vi "Library Path.vi"() -> (0 "Library Path":path=path "C:/LQ/bin/LQ.dll")   [LabVIEW 2014, in "LQ Core.lvlib"]
uses:
  LQ Core.lvlib
  <vilib>/Utility/sysdir.llb/System Directory Type.ctl
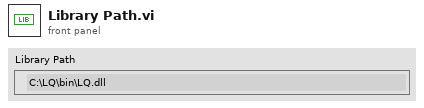
[diagram p1: front panel]
types:
  T1 = typedef "System Directory Type.ctl" = i32
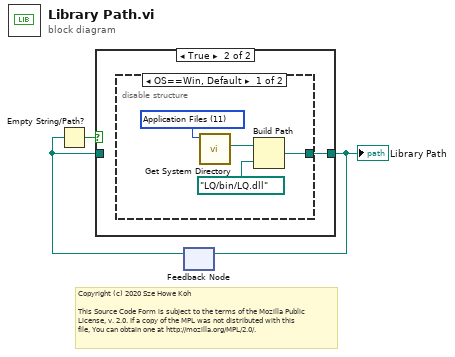
[diagram p0: block diagram]
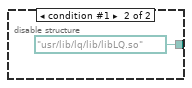
[diagram p3: hidden frame]
diagram:
  # "Copyright (c) 2020 Sze Howe Koh\n\nThis Source Code Form is subject to the terms of the Mozilla Public\nLicense, v. 2.0. If a copy of the MPL was not distributed with this\nfile, You can obtain one at http://mozilla.org/MPL/2.0/."
  n1 = feedback #1() -> (w2:path)  [unwired: 1 in]
  n2 = Empty String/Path?(string/path=w2) -> (empty?=w3:bool)
  n3 = case shown="True" w3 {
    tunnel: [w4 w5] -> w1
    tunnel: w2 -> [w4 _]
    frame False {
    }
    frame True {
      n4 = disable-structure shown="OS==Win, Default" {
        disable-tunnel: [w7 path "/usr/lib/lq/lib/libLQ.so" ("appended path")] -> w5
        frame condition #0 (active) {
          w8 = T1 11 items=["User Home"=0, "User Desktop"=1, "User Documents"=2, "User Application Data"=3, "User Preferences"=4, "User Temporary"=5, "Public Documents"=6, "Public Application Data"=7, "Public Preferences"=8, "Public Cache"=13, "System Core Libraries"=9, "System Installed Libraries"=10, "Application Files"=11, "Boot Volume Root"=12] ("system directory type")
          n5 = call <vilib>:"Get System Directory.vi"("system directory type"=w8) -> ("system directory"=w9:path)  [unwired: 10 in]
          n6 = Build Path(base path=w9, name or relative path=path "LQ/bin/LQ.dll") -> (appended path=w7:path)
        }
        frame condition #1 {
        }
      }
    }
  }
  "Library Path" <- w1
  n7 = feedback-in #1(w1) -> ()
